vi "Encode YAML.vi"() -> ()   [LabVIEW 2016]
uses:
  METADATA.ctl
  Components/YAML Parser.lvlib
panel:
  in  "Metadata Cluster":T1
  in  "Weight":dbl=80.0
  out "YAML String":string
  in  "Phones":string[](array[string])=["06.43.94.98.85", "06.43.94.98.86"]
  in  "Size":dbl=182.1
  in  "Male":bool=TRUE
  in  "Age":u32=27
  in  "Address":string="10 rue Jean Prévost\n38000 Grenoble\nFrance"
  in  "Name":string="Nicolas Bats"
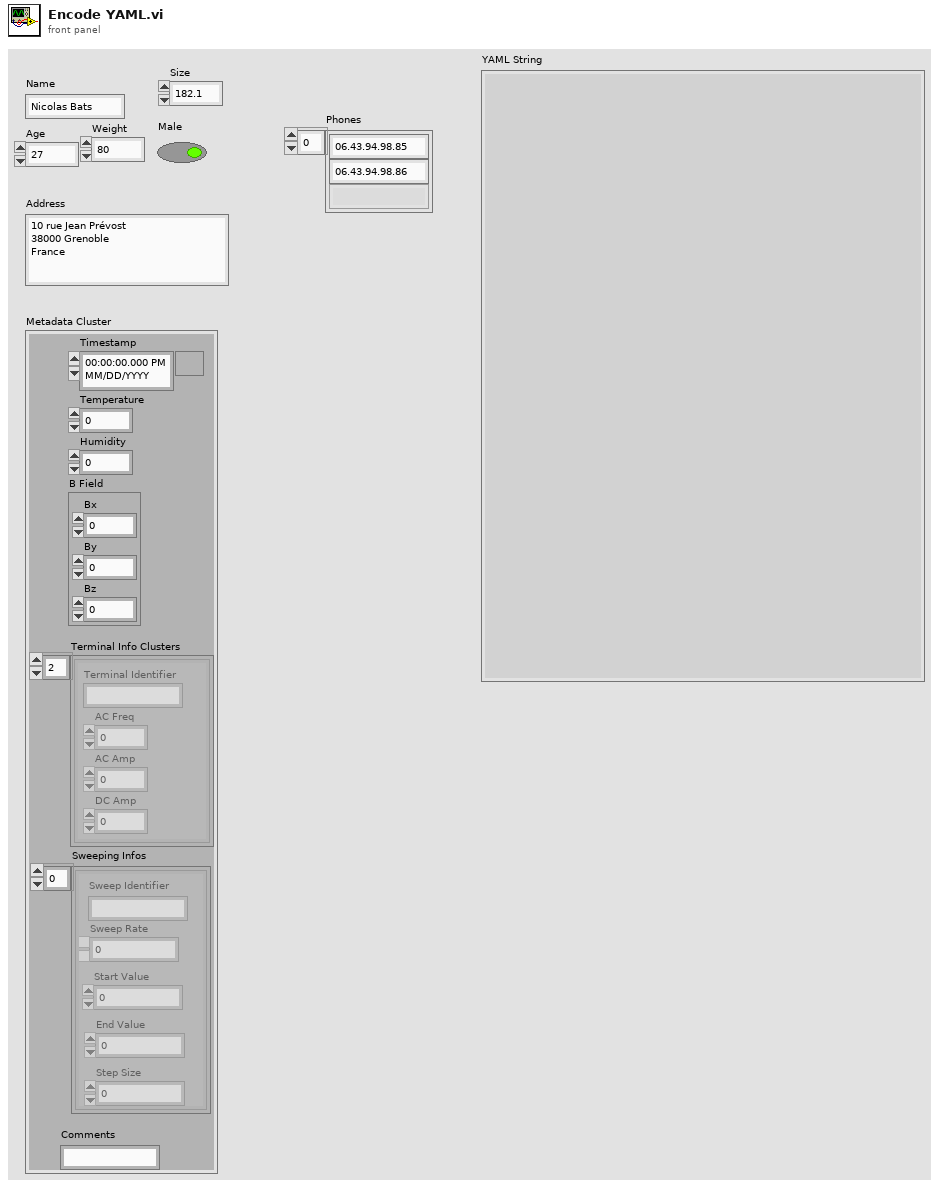
[diagram p1: front panel]
types:
  T1 = typedef "METADATA.ctl" = cluster{"Timestamp":timestamp, "Temperature":dbl, "Humidity":dbl, "B Field":cluster{"Bx":dbl, "By":dbl, "Bz":dbl}, "Terminal Info Clusters":cluster{"Terminal Identifier":string, "AC Freq":dbl, "AC Amp":dbl, "DC Amp":dbl}[], "Sweeping Infos":cluster{"Sweep Rate":dbl, "Sweep Identifier":string, "Start Value":dbl, "End Value":dbl, "Step Size":dbl}[], "Comments":string}
  T2 = cluster{"Male":bool, "Name":string, "Age":u32, "Physical":cluster{"Size":dbl, "Weight":dbl}, "Address":string, "Phones":string[], "seconds since 1Jan1904":timestamp}
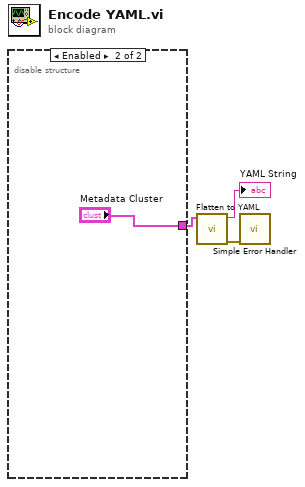
[diagram p0: block diagram]
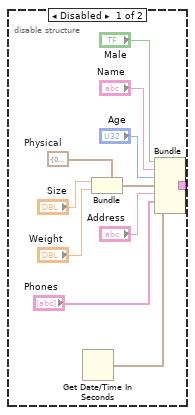
[diagram p2: hidden frame]
diagram:
  n1 = disable-structure shown="Enabled" {
    disable-tunnel: [w10 "Metadata Cluster"] -> w3
    frame Disabled {
      w6 = cluster{"Size":dbl, "Weight":dbl} {"Size"=0.0, "Weight"=0.0}  # Physical
      n2 = Get Date/Time In Seconds() -> (seconds since 1Jan1904=w4:timestamp)
      n3 = Bundle(cluster=w6, "Size"="Size", "Weight"="Weight") -> (w7:cluster{"Size":dbl, "Weight":dbl})
      n4 = Bundle("Male"="Male", "Name"="Name", "Age"="Age", "Physical"=w7, "Address"="Address", "Phones"="Phones", "seconds since 1Jan1904"=w4) -> (w10:T2)  [unwired: 1 in]
    }
    frame Enabled {
    }
  }
  n5 = call "Flatten to YAML.vi"("Anything"=w3) -> ("error out"=w2:errorcluster, "YAML String"=→"YAML String":string)  [unwired: 9 in]
  n6 = call <vilib>:"Simple Error Handler.vi"("error in (no error)"=w2) -> ()  [unwired: 4 in, 5 out]
